vi "Analog Functions.vi"(0 "System no.":i32=1 min=1 max=20 step=1, 1 "String to send":string, 3 "AI Task":refnum<k21>, 4 "AO Task":refnum<k21>, 5 "error in":errorcluster, 6 "Waveform to write":waveform(dbl)[](array[waveform]), 7 "Continuously?":bool=TRUE) -> (14 "String output":string, 15 "Boolean output":bool, 19 "error out":errorcluster)   [LabVIEW 2026]
doc: "This vi calls Analog Functions (dyn).vi functions dynamically during runtime, depending on \"String to send\". \n\nValid for Analog Systems (but must be present for all other systems, too)"
uses:
  Available Analog Commands.ctl
panel:
  out "Command":T1
  # "This vi calls Analog Functions (dyn).vi functions dynamically during runtime, depending on \n\"String to send\".  DUMMY VI!"
  # "General inputs:"
  # "Task IDs In"
  # "W_Wave settings:"
  # "Outputs:"
  # "Error handling:"
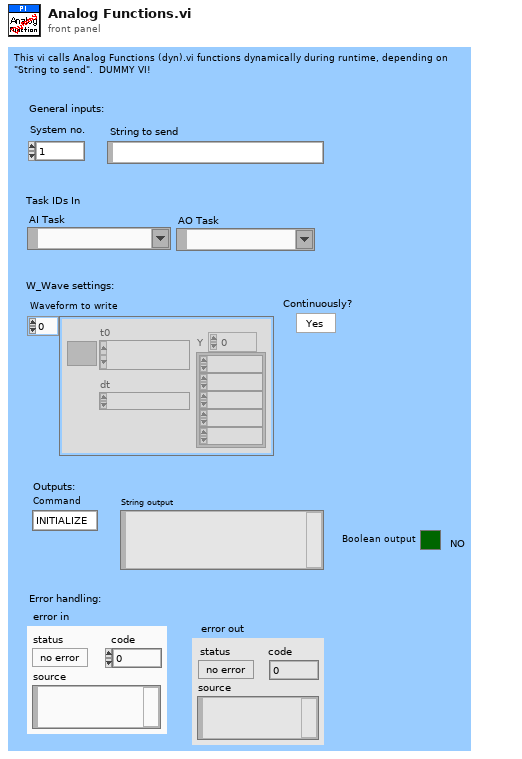
[diagram p1: front panel]
types:
  T1 = typedef "Available Analog Commands.ctl" = enum16{"INITIALIZE", "VOL?", "VOL ", "CLOSE", "MOV", "POS?", "VCO", "VCO?", "WAIT_WF", "TMN?", "TMX?", "VEL", "VEL?", "SAI?", "MVR", "ERR?", "#24", "STP", "*IDN?", "#5", "STE", "DRR?", "W_Wave", "HLP?", "W/R_Wave"}
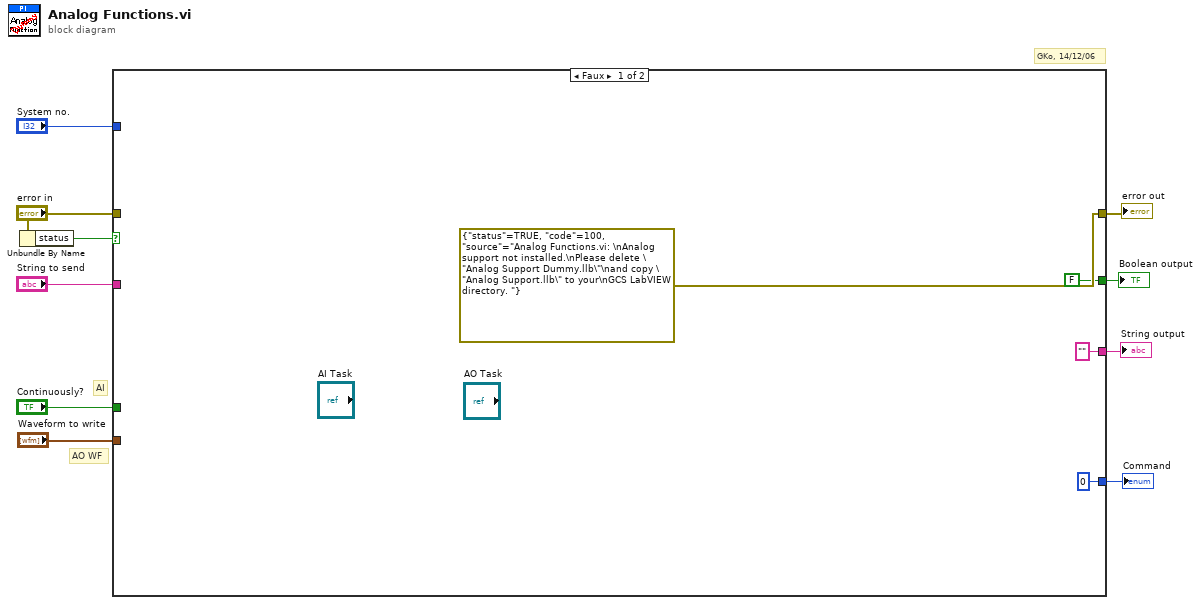
[diagram p0: block diagram]
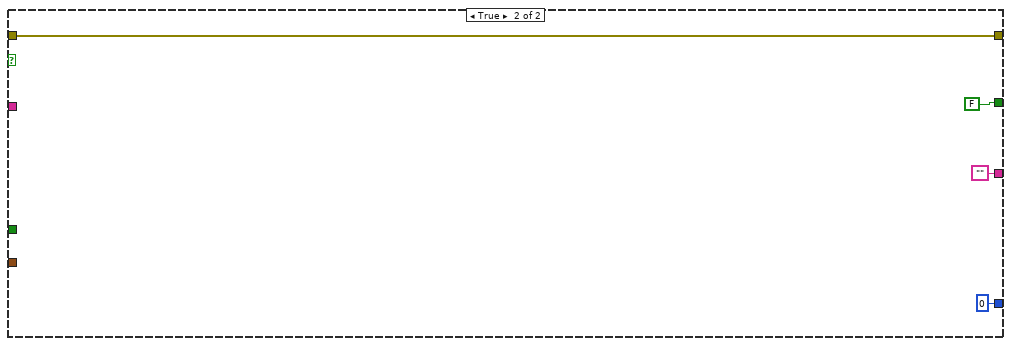
[diagram p2: hidden frame]
diagram:
  # "AI"
  # "AO WF"
  # "GKo, 14/12/06"
  n1 = Unbundle By Name("error in") -> ("status"=w9:bool)
  n2 = case shown="Faux" w9 {
    tunnel: [errorcluster {"status"=TRUE, "code"=100, "source"="Analog Functions.vi: \nAnalog support not installed.\nPlease delete \"Analog Support Dummy.llb\"\nand copy \"Analog Support.llb\" to your\nGCS LabVIEW directory. "} ("error in") w18] -> w8
    tunnel: "error in" -> [_ w18]
    tunnel: ["" ("szAnswer") "" ("szAnswer")] -> w7
    tunnel: "String to send" -> [_ _]
    tunnel: "System no." -> [_ _]
    tunnel: [FALSE ("Boolean output") FALSE ("Boolean output")] -> w4
    tunnel: [0 0] -> w3
    tunnel: "Continuously?" -> [_ _]
    tunnel: "Waveform to write" -> [_ _]
    frame False {
    }
    frame True {
    }
  }
  "error out" <- w8
  "String output" <- w7
  "Boolean output" <- w4
  "Command" <- w3
